vi "initial weights.vi"(2 "Number of classifiers":i32, 3 "Number of hidden neurons":i32, 4 "Inputs + 1":i32) -> (0 "Weights 2":dbl[][](array[numeric]), 1 "Weights 1":dbl[][](array[numeric]))   [LabVIEW 2009]
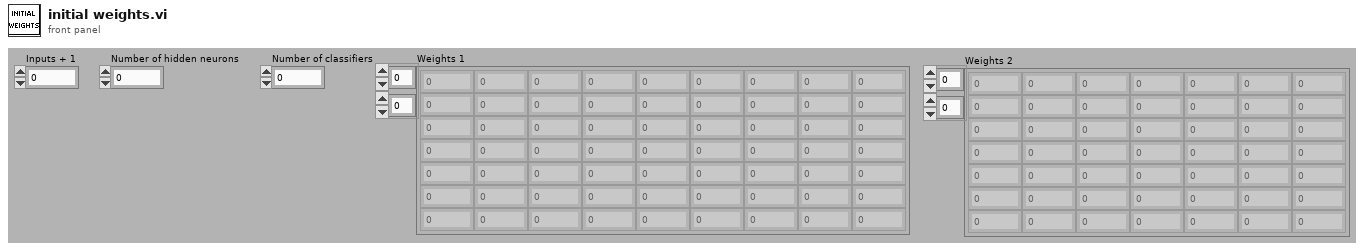
[diagram p1: front panel]
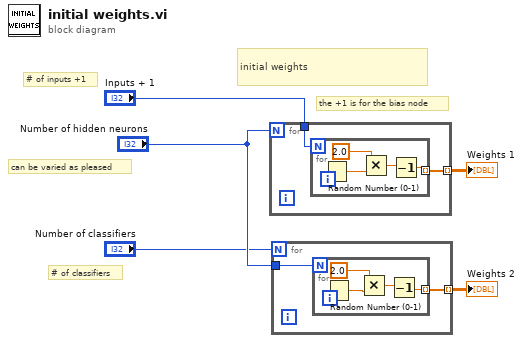
[diagram p0: block diagram]
diagram:
  # "# of classifiers"
  # "can be varied as pleased"
  # "# of inputs +1"
  # "the +1 is for the bias node"
  # "initial weights"
  n1 = for {
    N: "Number of hidden neurons" -> [_]
    tunnel: [w7] -> w3 mode=indexing
    tunnel: "Inputs + 1" -> [w6]
    n2 = for {
      N: w6 -> [_]
      tunnel: [w8] -> w7 mode=indexing
      n3 = Random Number (0-1)() -> (number: 0 to 1=w11:dbl)
      n4 = Multiply(x=2.0, y=w11) -> (x*y=w9:dbl)
      n5 = Decrement(x=w9) -> (x-1=w8:dbl)
    }
  }
  "Weights 1" <- w3
  n6 = for {
    N: "Number of classifiers" -> [_]
    tunnel: [w13] -> w4 mode=indexing
    tunnel: "Number of hidden neurons" -> [w12]
    n7 = for {
      N: w12 -> [_]
      tunnel: [w14] -> w13 mode=indexing
      n8 = Random Number (0-1)() -> (number: 0 to 1=w15:dbl)
      n9 = Multiply(x=2.0, y=w15) -> (x*y=w17:dbl)
      n10 = Decrement(x=w17) -> (x-1=w14:dbl)
    }
  }
  "Weights 2" <- w4
